vi "Global info.vi"() -> ()   [LabVIEW 2016]
panel:
  in  "Previous Button":bool
  # "Global Info"
  # "The International Space Station (ISS) is a space station, or a habitable artificial satellite, in low Earth orbit. Its first component launched into orbit in 1998, and the ISS is now the largest man-made body in low Earth orbit and can often be seen with the naked eye from Earth. The ISS consists of pressurised modules, external trusses, solar arrays, and other components. ISS components have been launched by Russian Proton and Soyuz rockets, and American Space Shuttles."
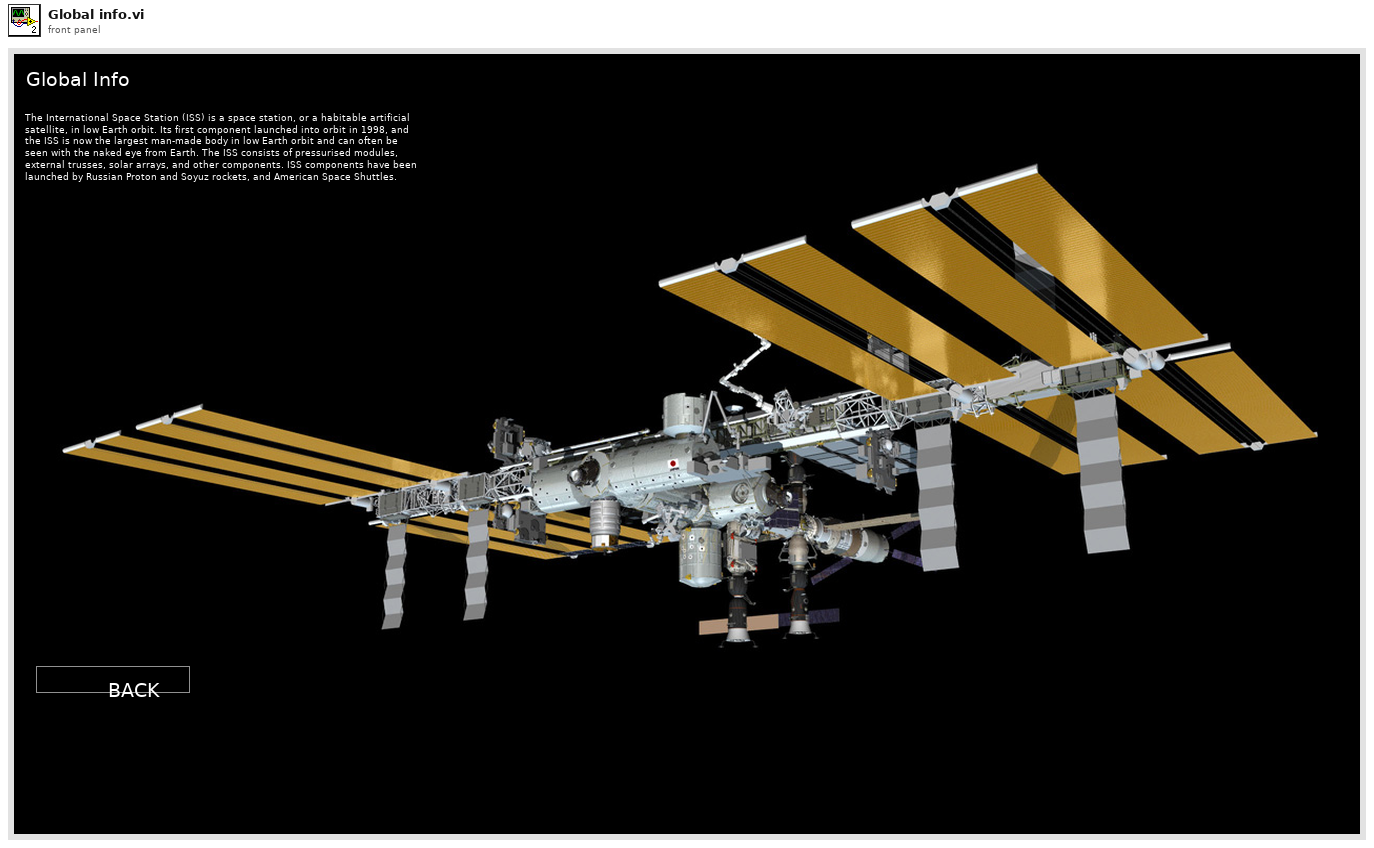
[diagram p1: front panel]
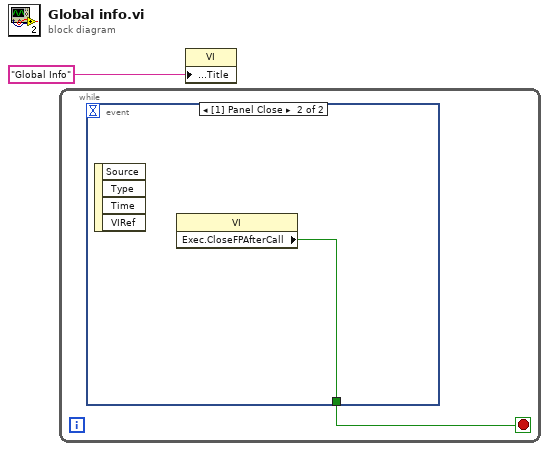
[diagram p0: block diagram]
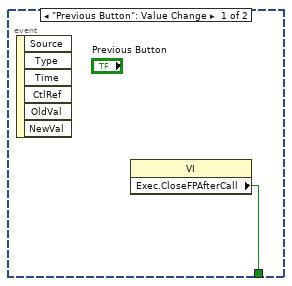
[diagram p2: hidden frame]
diagram:
  n1 = while {
    stop <- w2 stop-if-true
    n2 = event shown="[1] Panel Close" {
      selector: _ -> [_ _]
      dyn-events: _ -> [_ _]
      timeout: _ -> [_ _]
      tunnel: [w3 w4] -> w2
      event "Previous Button": Value Change {
        n3 = event-data() -> ()  [unwired: 1 in, 6 out]
        n4 = property class="VI"() -> ("Exec.CloseFPAfterCall"=w3:bool)  [unwired: 2 in, 2 out]
      }
      event Panel Close {
        n5 = event-data() -> ()  [unwired: 1 in, 4 out]
        n6 = property class="VI"() -> ("Exec.CloseFPAfterCall"=w4:bool)  [unwired: 2 in, 2 out]
      }
    }
  }
  n7 = property class="VI"("Front Panel.Title"="Global Info" ("Front Panel Window:Title")) -> ()  [unwired: 2 in, 2 out]
